vi "DestroyTopic.vi"(8 "error in (no error)":errorcluster, 10 "Topic Actor":string, 11 "Message Broker Interface TAP in":refnum<class "Message Broker Interface Ref.lvclass">) -> (0 "error out":errorcluster, 2 "Found?":bool, 3 "Message Broker Interface TAP out":refnum<class "Message Broker Interface Ref.lvclass">)   [LabVIEW 2016, in "Stream Mediator.lvlib" / "Message Broker Interface Ref.lvclass"]
doc: "--\nCopyright © 2017 Composed SystemsI All rights reserved.\n\nAuthor: Jon McBee <jon.mcbee@composed.io>\n\nThis library is provided \"AS IS\" ,WITHOUT WARRANTIES OR\nCONDITIONS OF ANY KIND, either express or implied.\n\nComposed Systems -- composed.io\n\nStream 0.0.1.1\nJon McBee - Composed Systems\nCopyright (c) 2017, Composed Systems"
uses:
  <userlib>/Composed Systems/Stream/Mediator/Classes/Message Broker Interface Ref/Message Broker Interface Ref.lvclass
  <userlib>/Composed Systems/Stream/Mediator/Classes/Message Broker Interface Ref/Message Broker Interface Ref.lvclass/Message Broker Interface Ref.ctl
  <userlib>/Composed Systems/Stream/Mediator/Classes/Message Broker/Message Broker.lvclass
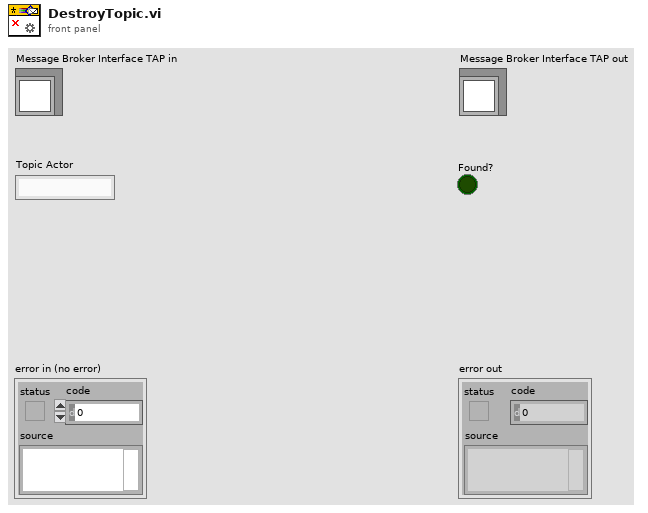
[diagram p1: front panel]
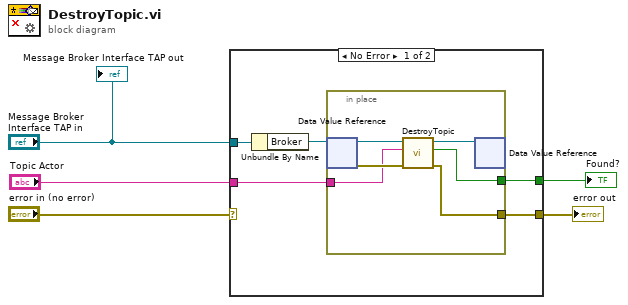
[diagram p0: block diagram]
diagram:
  n1 = case shown="No Error" "error in (no error)" {
    selector: "error in (no error)" -> [_ w17]
    tunnel: "Message Broker Interface TAP in" -> [w10 _]
    tunnel: [w8 w17] -> w3
    tunnel: "Topic Actor" -> [w7 _]
    tunnel: [w6 _] -> w1
    frame No Error {
      n2 = Unbundle By Name(w10) -> ("Broker"=w9:refnum<data-value>)
      n3 = in-place {
        in-place-border: [w13] -> w8
        in-place-border: w7 -> [w12]
        in-place-border: [w11] -> w6
        n4 = in-place-dvr #1(w9) -> (w16:refnum<class "Message Broker.lvclass">, w14:errorcluster)
        n5 = call <userlib>:"DestroyTopic.vi"("error in (no error)"=w14, "Topic Actor"=w12, "Message Broker in"=w16) -> ("error out"=w13:errorcluster, "Found?"=w11:bool, "Message Broker out"=w15:refnum<class "Message Broker.lvclass">)  [unwired: 6 in]
        n6 = in-place-dvr #1(w15) -> ()  [unwired: 2 out]
      }
    }
    frame Error {
    }
  }
  "error out" <- w3
  "Found?" <- w1
  "Message Broker Interface TAP out" <- "Message Broker Interface TAP in"
